vi "SetParam.vi"(8 "error in (no error)":errorcluster caption="entrée d'erreur (pas d'erreur)", 10 "PowerTransformer":T1={"method"="yeo-johnson", "standardize"=TRUE, "copy"=TRUE}, 11 "PowerTransformer.lvclass":refnum<class "PowerTransformer.lvclass">) -> (0 "error out":errorcluster caption="sortie d'erreur", 3 "PowerTransformer.lvclass":refnum<class "PowerTransformer.lvclass">)   [LabVIEW 2020, in "PowerTransformer.lvclass"]
doc: "Set Parameters"
uses:
  PowerTransformer.lvclass
  PowerTransformer.lvclass/PowerTransformer.ctl
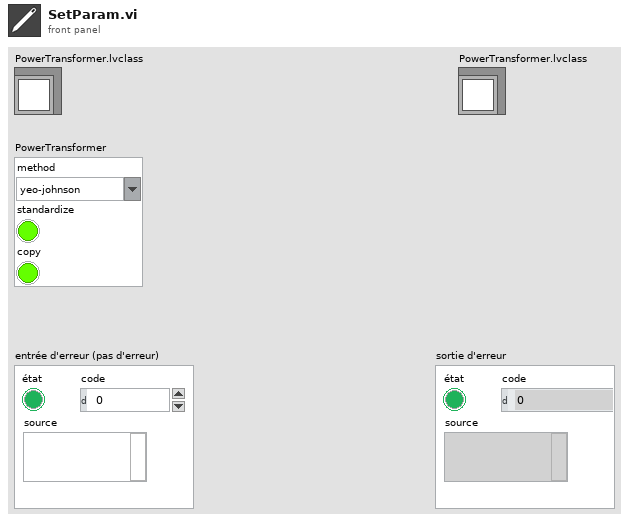
[diagram p1: front panel]
types:
  T1 = cluster{"method":string, "standardize":bool, "copy":bool}
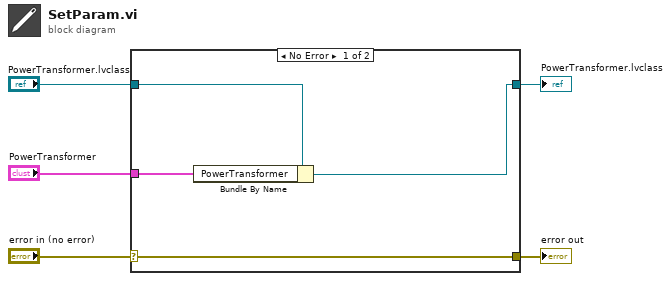
[diagram p0: block diagram]
diagram:
  n1 = case shown="No Error" "error in (no error)" {
    selector: "error in (no error)" -> [w9 w10]
    tunnel: [w9 w10] -> w4
    tunnel: [w7 w11] -> w2
    tunnel: "PowerTransformer.lvclass" -> [w8 w11]
    tunnel: "PowerTransformer" -> [w6 _]
    frame No Error {
      n2 = Bundle By Name(cluster=w8, "PowerTransformer"=w6) -> (w7:refnum<class "PowerTransformer.lvclass">)
    }
    frame Error {
    }
  }
  "error out" <- w4
  "PowerTransformer.lvclass" <- w2
